vi "HW Match Status.vi"(8 "error in (no error)":errorcluster, 10 "Pass (F) / Fail (T)":bool, 11 "FP Controls in":refnum<class "FP Controls.lvclass">) -> (0 "error out":errorcluster, 3 "FP Controls out":refnum<class "FP Controls.lvclass">)   [LabVIEW 2012, in "Configuration Grandmaster.lvlib" / "FP Controls.lvclass"]
uses:
  FP Controls.lvclass
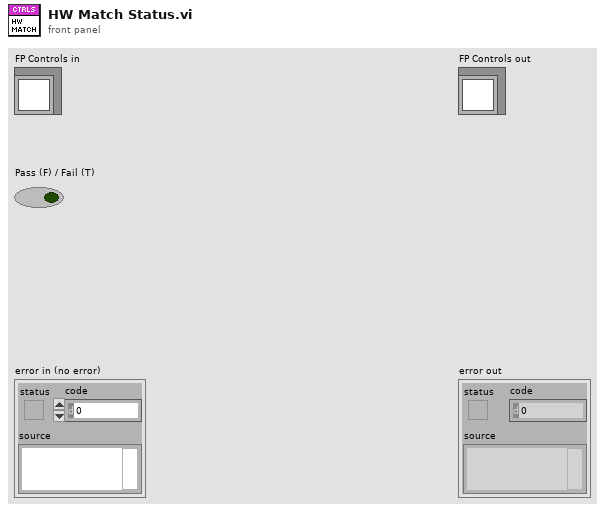
[diagram p1: front panel]
types:
  T1 = enum8{"Enabled", "Disabled", "Disabled and Grayed Out"}
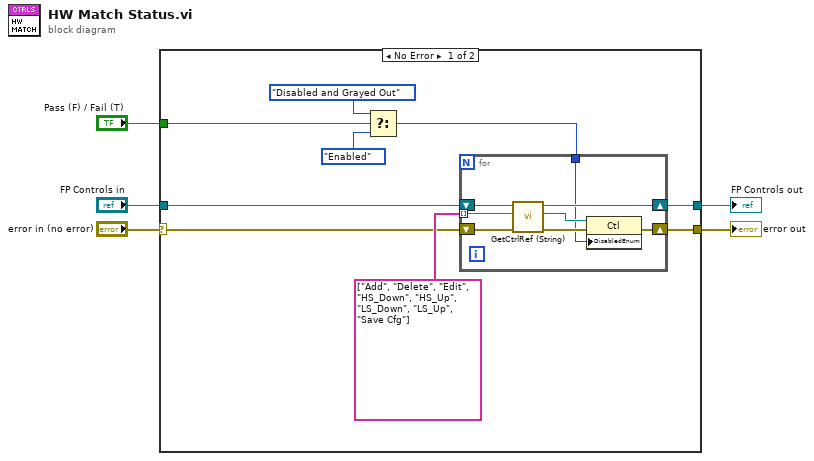
[diagram p0: block diagram]
diagram:
  n1 = case shown="No Error" "error in (no error)" {
    selector: "error in (no error)" -> [w7 w24]
    tunnel: [w6 w24] -> w4
    tunnel: [w9 w23] -> w2
    tunnel: "FP Controls in" -> [w10 w23]
    tunnel: "Pass (F) / Fail (T)" -> [w14 _]
    frame No Error {
      n2 = Select(t=T1."Disabled and Grayed Out" ("Disabled"), s=w14, f=T1."Enabled" ("Disabled")) -> (s? t:f=w8:T1)
      n3 = for {
        shift-right: [w17] -> w6
        shift-left: w7 -> [w21]
        tunnel: string[] ["Add", "Delete", "Edit", "HS_Down", "HS_Up", "LS_Down", "LS_Up", "Save Cfg"] -> [w20] mode=indexing
        shift-right: [w16] -> w9
        shift-left: w10 -> [w22]
        tunnel: w8 -> [w15]
        n4 = call "GetCtrlRef (String).vi"("error in (no error)"=w21, "FP Control"=w20, "FP Controls in"=w22) -> ("error out"=w19:errorcluster, "Ctrl Ref"=w18:refnum<vi>, "FP Controls out"=w16:refnum<class "FP Controls.lvclass">)  [unwired: 6 in]
        n5 = property class="Ctl"(reference=w18, error in=w19, "DisabledEnum"=w15) -> (error out=w17:errorcluster)  [unwired: 1 out]
      }
    }
    frame Error {
    }
  }
  "error out" <- w4
  "FP Controls out" <- w2
